vi "TEST.vi"(8 "error in (no error)":errorcluster) -> (0 "error out":errorcluster)   [LabVIEW 2017]
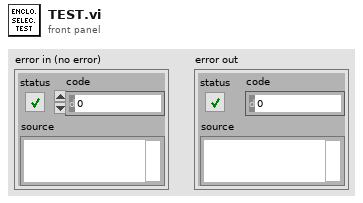
[diagram p1: front panel]
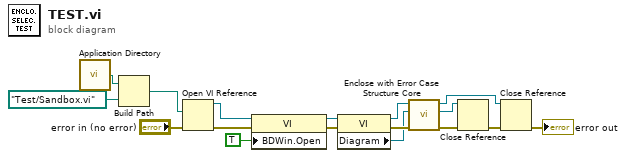
[diagram p0: block diagram]
diagram:
  n1 = call <vilib>:"Application Directory.vi"() -> ("Application Directory"=w16:path)
  n2 = Build Path(base path=w16, name or relative path=path "Test/Sandbox.vi") -> (appended path=w17:path)
  n3 = Open VI Reference(vi path=w17, error in (no error)="error in (no error)") -> (vi reference=w14:refnum<vi>, error out=w15:errorcluster)  [unwired: 4 in]
  n4 = property on="Property Node" class="VI"(reference=w14, error in=w15, "BDWin.Open"=TRUE ("Front Panel Window:Open")) -> (reference out=w8:refnum<vi>, error out=w12:errorcluster)
  n5 = property class="VI"(reference=w8, error in=w12) -> (reference out=w9:refnum<vi>, error out=w11:errorcluster, "Diagram"=w10:refnum<vi>)
  n6 = call "Enclose with Error Case Structure Core.vi"("error in (no error)"=w11, "block diagram in"=w10, "VI in"=w9) -> ("error out"=w6:errorcluster, "block diagram out"=w4:refnum<vi>, "VI out"=w2:refnum<vi>)  [unwired: 6 in]
  n7 = Close Reference(reference=w4, error in (no error)=w6) -> (error out=w5:errorcluster)
  n8 = Close Reference(reference=w2, error in (no error)=w5) -> (error out=→"error out":errorcluster)
